vi "Tosca-Restore Visual Display Settings.vi"() -> (8 "Visual Display Settings":T1={"Use PTB"=TRUE, "IP Address"="localhost", "Port"=4926, "rect"={"left"=0, "top"=0, "width"=800, "height"=480}, "Full screen"=TRUE, "Open at start"=FALSE, "Monitor"=2, "Monitor size (in)"=8.0, "Monitor dist (in)"=24.0, "Photodiode Square"={"size"=50, "location"=enum."Bottom Left"}, "Background"=0.0}, 15 "error out":errorcluster)   [LabVIEW 2020]
uses:
  Tosca-Visual Display Settings.ctl
  Sub VIs/Tosca-Globals.vi
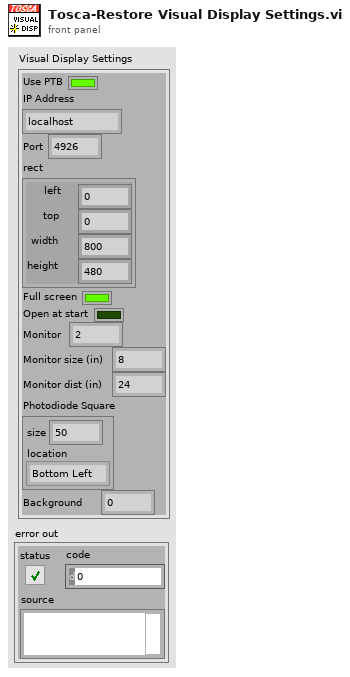
[diagram p1: front panel]
types:
  T1 = typedef "Tosca-Visual Display Settings.ctl" = cluster{"Use PTB":bool, "IP Address":string, "Port":i32, "rect":cluster{"left":i16, "top":i16, "width":i16, "height":i16}, "Full screen":bool, "Open at start":bool, "Monitor":i32, "Monitor size (in)":dbl, "Monitor dist (in)":dbl, "Photodiode Square":cluster{"size":i16, "location":enum16{"Bottom Left", "Top Left", "Top Right", "Bottom Right"}}, "Background":dbl}
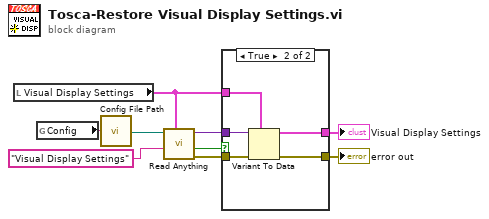
[diagram p0: block diagram]
diagram:
  n1 = local read "Visual Display Settings"() -> (w4:T1)
  n2 = global read "Tosca-Globals.vi" "Config"() -> (w1:string)
  n3 = call "Config File Path.vi"("AppName"=w1) -> ("Default config file name"=w9:path)
  n4 = call "Read Anything.vi"("Type of Anything"=w4, "Section Name (Name of \"Type of Anything\")"="Visual Display Settings" ("Section Name (Name of \"Type of Anything\")"), "Path (dialog)"=w9) -> ("Error Out"=w5:errorcluster, "Found?"=w7:bool, "Anything"=w6:variant)  [unwired: 6 in]
  n5 = case shown="True" w7 {
    tunnel: w6 -> [_ w15]
    tunnel: w5 -> [w10 w16]
    tunnel: w4 -> [w11 w14]
    tunnel: [w11 w13] -> w3
    tunnel: [w10 w12] -> w2
    frame False {
    }
    frame True {
      n6 = Variant To Data(error in=w16, type=w14, Variant=w15) -> (data=w13:T1, error out=w12:errorcluster)
    }
  }
  "Visual Display Settings" <- w3
  "error out" <- w2
